vi "RS485.vi"(0 "ModbusIn":T1, 3 "error in":errorcluster) -> (7 "ValoresLidos":u16[](array[numeric]), 10 "error out":errorcluster)   [LabVIEW 2019]
uses:
  TelaConfig/Configuracao.Variaveis.vi
  <vilib>/NI/Modbus Library/API/Wrapper/Create Serial Master.vi
  <vilib>/NI/Modbus Library/API/Master/Modbus Master.lvclass
  <vilib>/NI/Modbus Library/API/Wrapper/API Main.lvlib
  <vilib>/NI/Modbus Library/API/Slave/Modbus Slave.lvclass
panel:
  in  "Manual":bool
  in  "EndereçoSerial(1)":u8=1
  in  "TaxaComunicSerial":u32=9600
  in  "Paridade(even)":u16(ring)=2 items=["None", "Odd", "Even", "Mark", "Space"]
  in  "ComPort":refnum<visa-resource-name>
  out "number":u32
  out "BooleanLidos":bool[](array[boolean])
  out "Valor":u16
  in  "Stop Button":bool
  out "Bool sinais":bool[](array[boolean])
  out "ErrorAntesFechaCOM":errorcluster
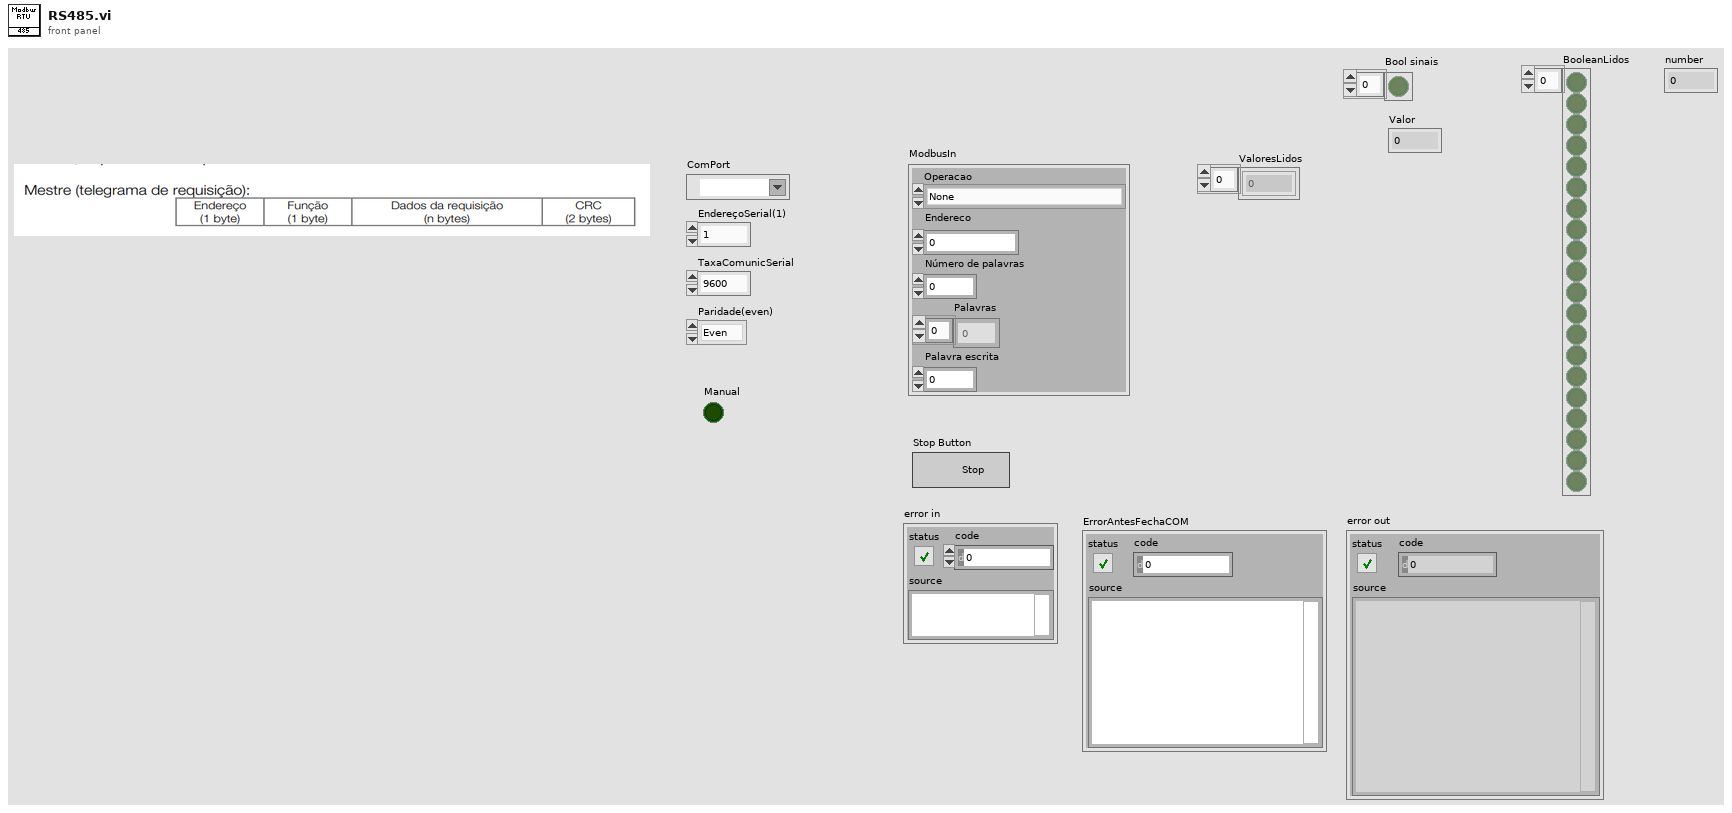
[diagram p1: front panel]
types:
  T1 = cluster{"Operacao":enum16{"None", "Read Input Registers VI", "Read Discrete Inputs VI", "Read Holding Registers VI", "Read Coils VI", "Write Multiple Holding Registers", "Write Multiple Input Registers ", "Write Single Holding Registers"}, "Endereco":u16, "Número de palavras":u16, "Palavras":u16[], "Palavra escrita":u16}
  T2 = enum16{"None", "Read Input Registers VI", "Read Discrete Inputs VI", "Read Holding Registers VI", "Read Coils VI", "Write Multiple Holding Registers", "Write Multiple Input Registers ", "Write Single Holding Registers"}
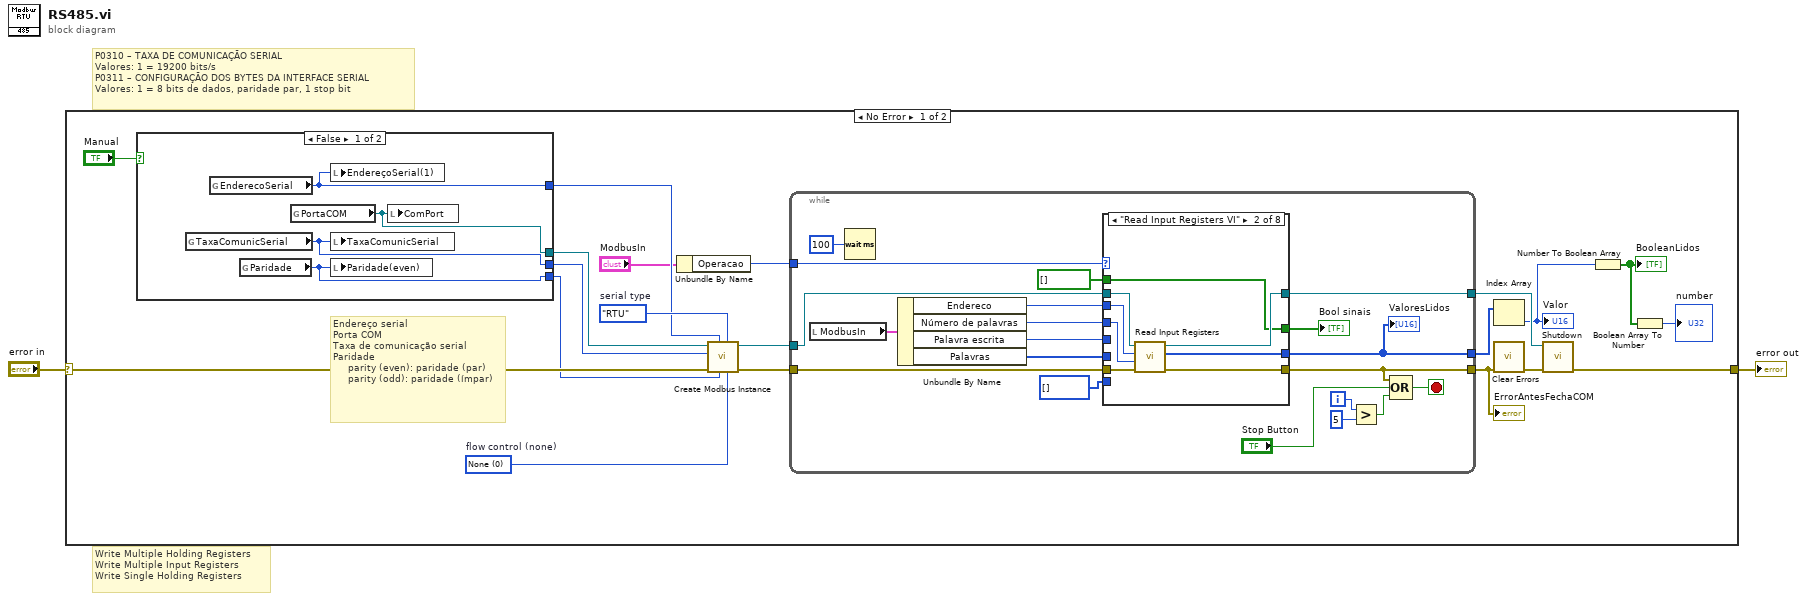
[diagram p0: block diagram]
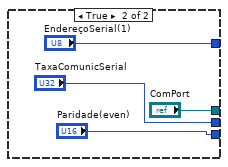
[diagram p2: hidden frame]
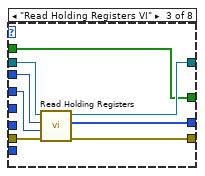
[diagram p4: hidden frame]
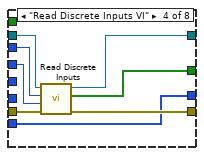
[diagram p5: hidden frame]
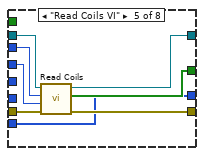
[diagram p6: hidden frame]
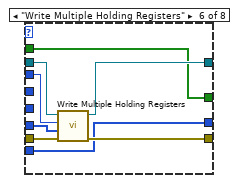
[diagram p7: hidden frame]
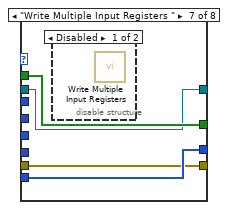
[diagram p8: hidden frame]
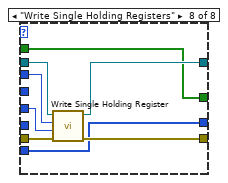
[diagram p10: hidden frame]
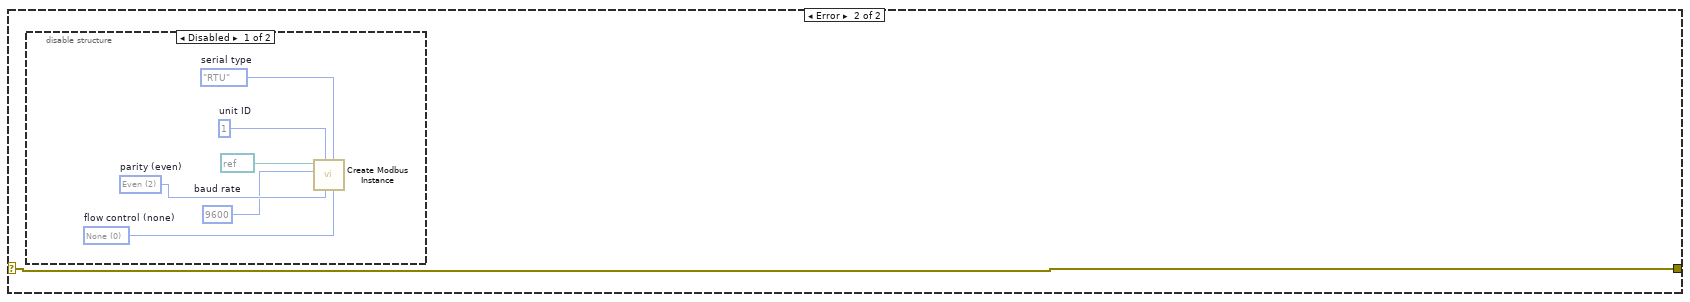
[diagram p11: hidden frame]
diagram:
  # "Write Multiple Holding Registers \nWrite Multiple Input Registers \nWrite Single Holding Registers"
  # "P0310 – TAXA DE COMUNICAÇÃO SERIAL \nValores: 1 = 19200 bits/s\nP0311 – CONFIGURAÇÃO DOS BYTES DA INTERFACE SERIAL \nValores: 1 = 8 bits de dados, paridade par, 1 stop bit"
  n1 = case shown="No Error" "error in" {
    selector: "error in" -> [w21 w107]
    tunnel: [w20 w107] -> w1
    frame No Error {
      w18 = u16 0 items=["None", "XON/XOFF", "RTS/CTS", "XON/XOFF & RTS/CTS", "DTR/DSR", "XON/XOFF & DTR/DSR"]  # flow control (none)
      w19 = enum16{"RTU", "ASCII"}."RTU"  # serial type
      # "Endereço serial\nPorta COM \nTaxa de comunicação serial\nParidade\n     parity (even): paridade (par)\n     parity (odd): paridade (ímpar)"
      n2 = case shown="False" "Manual" {
        tunnel: [w25 "ComPort"] -> w22
        tunnel: [w26 "EndereçoSerial(1)"] -> w8
        tunnel: [w24 "TaxaComunicSerial"] -> w7
        tunnel: [w23 "Paridade(even)"] -> w6
        frame False {
          n3 = global read "Configuracao.Variaveis.vi" "TaxaComunicSerial"() -> (w24:u32)
          n4 = global read "Configuracao.Variaveis.vi" "EnderecoSerial"() -> (w26:u8)
          n5 = global read "Configuracao.Variaveis.vi" "Paridade"() -> (w23:u16)
          n6 = global read "Configuracao.Variaveis.vi" "PortaCOM"() -> (w25:refnum<visa-resource-name>)
          n7 = local write "EndereçoSerial(1)"(w26) -> ()
          n8 = local write "TaxaComunicSerial"(w24) -> ()
          n9 = local write "Paridade(even)"(w23) -> ()
          n10 = local write "ComPort"(w25) -> ()
        }
        frame True {
        }
      }
      n11 = Unbundle By Name("ModbusIn") -> ("Operacao"=w3:T2)
      n12 = call-poly <vilib>:"Create Modbus Instance.vi"("flow control (none)"=w18, "serial type"=w19, "parity (even)"=w6, "unit ID"=w8, "error in"=w21, "baud rate"=w7, "VISA resource name"=w22) -> ("error out"=w16:errorcluster, "serial master instance"=w17:refnum<class "Modbus Master.lvclass">)  [unwired: 3 in]
      n13 = while {
        tunnel: w17 -> [w48]
        tunnel: w16 -> [w47]
        tunnel: [w45] -> w15
        tunnel: [w46] -> w14
        tunnel: w3 -> [w41]
        tunnel: [w36] -> w12
        i -> [w44]
        stop <- w49 stop-if-true
        n14 = local read "ModbusIn"() -> (w35:T1)
        n15 = Wait (ms)(milliseconds to wait=u32 100) -> ()  [unwired: 1 out]
        n16 = Unbundle By Name(w35) -> ("Endereco"=w34:u16, "Número de palavras"=w33:u16, "Palavra escrita"=w32:u16, "Palavras"=w31:u16[])
        n17 = case shown="\"Read Input Registers VI\"" w41 {
          tunnel: w48 -> [w51 w61 w70 w78 w86 w90 w96 w106]
          tunnel: w34 -> [_ w60 w69 w77 w85 w94 _ w102]
          tunnel: w33 -> [_ w59 w68 w76 w84 _ _ _]
          tunnel: w47 -> [w52 w62 w67 w75 w83 w93 w95 w103]
          tunnel: [w51 w58 w66 w74 w82 w91 w96 w105] -> w46
          tunnel: [w52 w56 w64 w72 w81 w92 w95 w104] -> w45
          tunnel: [w54 w57 w65 w71 w79 w89 w98 w101] -> w36
          tunnel: [w53 w55 w63 w73 w80 w88 w97 w100] -> w40
          tunnel: u16[] [] ("register values") -> [w54 _ _ w71 w79 w89 w98 w101]
          tunnel: bool[] [] ("register values") -> [w53 w55 w63 _ _ w88 w97 w100]
          tunnel: w32 -> [_ _ _ _ _ _ _ w99]
          tunnel: w31 -> [_ _ _ _ _ w87 _ _]
          frame "None", Default {
          }
          frame "Read Input Registers VI" {
            n18 = call-dynamic "Read Input Registers.vi"("error in"=w62, "number of inputs"=w59, "starting address"=w60, "Modbus master in"=w61) -> ("error out"=w56:errorcluster, "register values"=w57:u16[], "Modbus master out"=w58:refnum<class "Modbus Master.lvclass">)  [unwired: 5 in]
          }
          frame "Read Holding Registers VI" {
            n19 = call-dynamic "Read Holding Registers.vi"("error in"=w67, "number of inputs"=w68, "starting address"=w69, "Modbus master in"=w70) -> ("error out"=w64:errorcluster, "register values"=w65:u16[], "Modbus master out"=w66:refnum<class "Modbus Master.lvclass">)  [unwired: 5 in]
          }
          frame "Read Discrete Inputs VI" {
            n20 = call-dynamic "Read Discrete Inputs.vi"("error in"=w75, "number of inputs"=w76, "starting address"=w77, "Modbus master in"=w78) -> ("error out"=w72:errorcluster, "discrete inputs"=w73:bool[], "Modbus master out"=w74:refnum<class "Modbus Master.lvclass">)  [unwired: 5 in]
          }
          frame "Read Coils VI" {
            n21 = call-dynamic "Read Coils.vi"("error in"=w83, "number of inputs"=w84, "starting address"=w85, "Modbus master in"=w86) -> ("error out"=w81:errorcluster, "coils"=w80:bool[], "Modbus master out"=w82:refnum<class "Modbus Master.lvclass">)  [unwired: 5 in]
          }
          frame "Write Multiple Holding Registers" {
            n22 = call-dynamic "Write Multiple Holding Registers.vi"("error in"=w93, "registers to write"=w87, "starting address"=w94, "Modbus master in"=w90) -> ("error out"=w92:errorcluster, "Modbus master out"=w91:refnum<class "Modbus Master.lvclass">)  [unwired: 6 in]
          }
          frame "Write Multiple Input Registers " {
            n23 = disable-structure shown="Disabled" {
              frame Disabled {
                n24 = call-dynamic "Write Multiple Input Registers.vi"() -> ()  [unwired: 10 in, 2 out]
              }
              frame Enabled {
              }
            }
          }
          frame "Write Single Holding Registers" {
            n25 = call-dynamic "Write Single Holding Register.vi"("error in"=w103, "register to write"=w99, "address"=w102, "Modbus master in"=w106) -> ("error out"=w104:errorcluster, "Modbus master out"=w105:refnum<class "Modbus Master.lvclass">)  [unwired: 6 in]
          }
        }
        "ValoresLidos" <- w36
        "Bool sinais" <- w40
        n26 = Greater?(x=w44, y=5) -> (0:w42:bool)
        n27 = Compound Arithmetic op=OR(w45, "Stop Button", w42) -> (w49:bool)
      }
      "ErrorAntesFechaCOM" <- w15
      n28 = Index Array(array=w12) -> (element=w11:u16)  [unwired: 1 in]
      "Valor" <- w11
      n29 = call <vilib>:"Clear Errors.vi"("error in (no error)"=w15) -> ("error out"=w13:errorcluster)  [unwired: 5 in, 1 out]
      n30 = call-dynamic "Shutdown.vi"("error in"=w13, "Modbus master in"=w14) -> ("error out"=w20:errorcluster)  [unwired: 9 in]
      n31 = Number To Boolean Array(number=w11) -> (Boolean array=w10:bool[])
      "BooleanLidos" <- w10
      n32 = Boolean Array To Number(Boolean array=w10) -> (number=→"number":u32)
    }
    frame Error {
      n33 = disable-structure shown="Disabled" {
        frame Disabled {
          w113 = u16 0 items=["None", "XON/XOFF", "RTS/CTS", "XON/XOFF & RTS/CTS", "DTR/DSR", "XON/XOFF & DTR/DSR"]  # flow control (none)
          w111 = u16 2 items=["None", "Odd", "Even", "Mark", "Space"]  # parity (even)
          w109 = u32 9600  # baud rate
          w112 = enum16{"RTU", "ASCII"}."RTU"  # serial type
          w110 = u8 1  # unit ID
          n34 = call-poly <vilib>:"Create Modbus Instance.vi"("flow control (none)"=w113, "serial type"=w112, "parity (even)"=w111, "unit ID"=w110, "baud rate"=w109, "VISA resource name"=refnum<visa-resource-name> refnum ("ComPort")) -> ()  [unwired: 4 in, 2 out]
        }
        frame Enabled {
        }
      }
    }
  }
  "error out" <- w1
